vi "Assert 2D Array wired to 2D Array Type.vi"   [LabVIEW 2017]
uses:
  3571a964-22ba-42f2-8cf4-bc27dbb6cb0e.vi
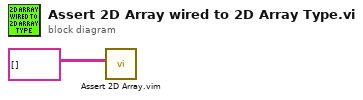
[diagram p0: block diagram]
diagram:
  n1 = call "Assert 2D Array.vim"("Array in"=string[][] []) -> ()  [unwired: 10 in, 1 out]
